vi "tm423_dualcamerasync.vi"() -> ()   [LabVIEW 2019]
panel:
  out "Camera Model":string
  out "Image":u16[][](graph)
  in  "capture":bool
  in  "Quit":bool
  out "Error Out":errorcluster {"code" format="%.0x"}
  # "This is an example of one way\nto synchronize two of the same\nmodel cameras."
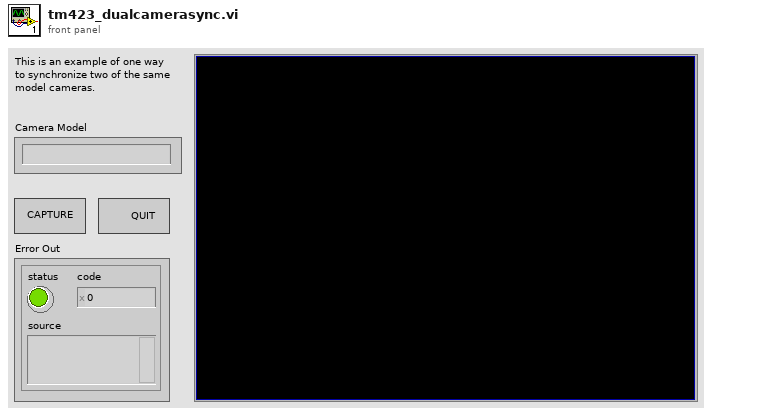
[diagram p1: front panel]
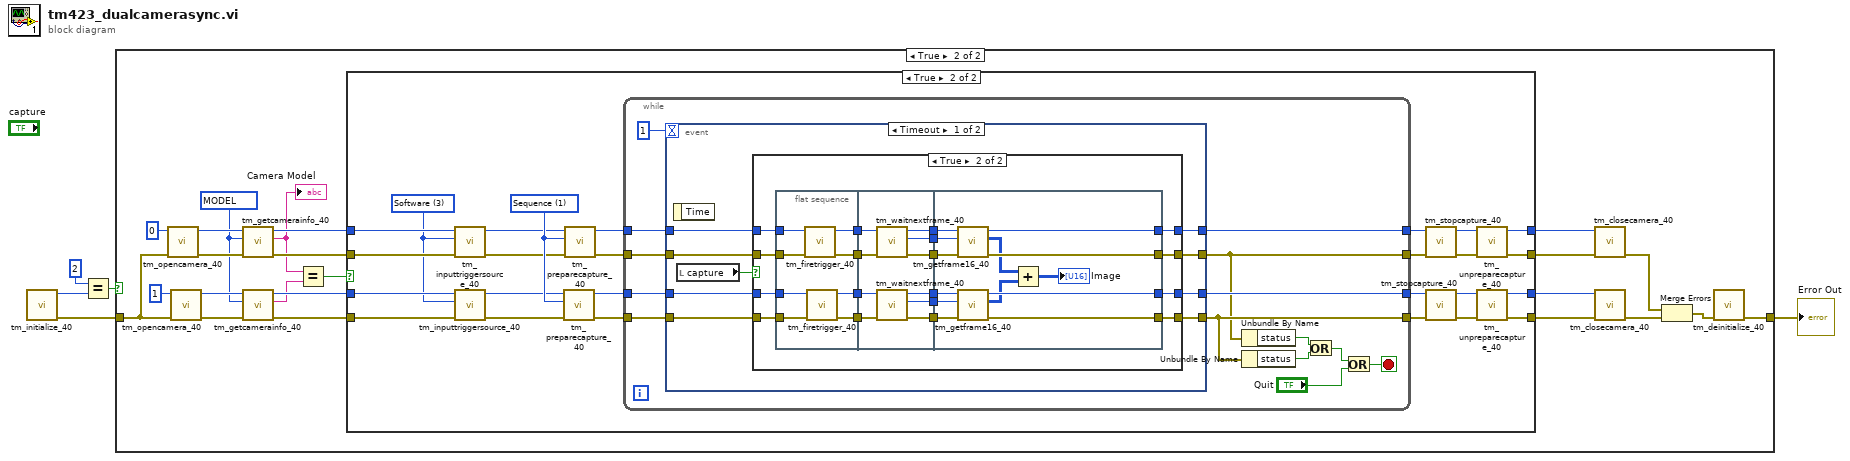
[diagram p0: block diagram]
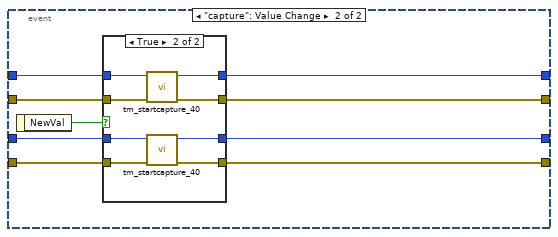
[diagram p5: hidden frame]
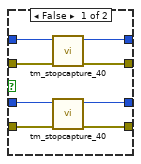
[diagram p6: hidden frame]
diagram:
  n1 = call <userlib>:"tm_initialize_40.vi"() -> ("error out"=w4:errorcluster, "Number Of Cameras"=w3:u32)  [unwired: 8 in, 2 out]
  n2 = Equal?(x=u32 2, y=w3) -> (x = y?=w1:bool)
  n3 = case shown="True" w1 {
    tunnel: w4 -> [w6 w26]
    tunnel: [w6 w28] -> w5
    frame False {
    }
    frame True {
      w18 = u32 67109124 items=["BUS"=67109121, "CAMERA ID"=67109122, "VENDOR"=67109123, "MODEL"=67109124, "CAMERA VERSION"=67109125, "DRIVER VERSION"=67109126, "MODULE VERSIOIN"=67109127, "DCAMAPI VERSION"=67109128] ("Info ID")
      n4 = call <userlib>:"tm_opencamera_40.vi"("error in (no error)"=w26, "Camera Index"=u32 0) -> ("error out"=w21:errorcluster, "Handle out"=w22:u32)  [unwired: 7 in, 1 out]
      n5 = call <userlib>:"tm_opencamera_40.vi"("error in (no error)"=w26, "Camera Index"=u32 1) -> ("error out"=w19:errorcluster, "Handle out"=w20:u32)  [unwired: 7 in, 1 out]
      n6 = call <userlib>:"tm_getcamerainfo_40.vi"("error in (no error)"=w21, "Info ID"=w18, "Handle in"=w22) -> ("error out"=w15:errorcluster, "String"=w9:string, "Handle out"=w14:u32)  [unwired: 6 in]
      "Camera Model" <- w9
      n7 = call <userlib>:"tm_getcamerainfo_40.vi"("error in (no error)"=w19, "Info ID"=w18, "Handle in"=w20) -> ("error out"=w16:errorcluster, "String"=w8:string, "Handle out"=w17:u32)  [unwired: 6 in]
      n8 = Equal?(x=w9, y=w8) -> (x = y?=w7:bool)
      n9 = case shown="True" w7 {
        tunnel: w17 -> [w33 w38]
        tunnel: w16 -> [w32 w37]
        tunnel: w15 -> [w31 w42]
        tunnel: w14 -> [w30 w41]
        tunnel: [w33 w50] -> w13
        tunnel: [w32 w49] -> w12
        tunnel: [w31 w47] -> w11
        tunnel: [w30 w48] -> w10
        frame False {
        }
        frame True {
          w34 = 3 items=["Internal"=1, "External"=2, "Software"=3, "Master Pulse"=4] ("Source")
          w51 = 1 items=["Snap", "Sequence"] ("Capture mode")
          n10 = call <userlib>:"tm_inputtriggersource_40.vi"("error in (no error)"=w42, "Source"=w34, "Handle in"=w41) -> ("error out"=w39:errorcluster, "Handle out"=w40:u32)  [unwired: 7 in]
          n11 = call <userlib>:"tm_inputtriggersource_40.vi"("error in (no error)"=w37, "Source"=w34, "Handle in"=w38) -> ("error out"=w35:errorcluster, "Handle out"=w36:u32)  [unwired: 7 in]
          n12 = call <userlib>:"tm_preparecapture_40.vi"("error in (no error)"=w35, "Capture mode"=w51, "Handle in"=w36) -> ("error out"=w43:errorcluster, "Handle out"=w44:u32)  [unwired: 5 in, 2 out]
          n13 = call <userlib>:"tm_preparecapture_40.vi"("error in (no error)"=w39, "Capture mode"=w51, "Handle in"=w40) -> ("error out"=w46:errorcluster, "Handle out"=w45:u32)  [unwired: 5 in, 2 out]
          n14 = while {
            tunnel: [w71] -> w59
            tunnel: [w65] -> w58
            tunnel: w44 -> [w73]
            tunnel: w43 -> [w72]
            tunnel: w45 -> [w68]
            tunnel: w46 -> [w67]
            tunnel: [w64] -> w52
            tunnel: [w66] -> w53
            stop <- w62 stop-if-true
            n15 = event shown="[0] Timeout" {
              selector: _ -> [_ _]
              dyn-events: _ -> [_ _]
              timeout: 1 -> [_ _]
              tunnel: w73 -> [w79 w143]
              tunnel: w72 -> [w78 w142]
              tunnel: [w75 w141] -> w71
              tunnel: [w74 w140] -> w65
              tunnel: w68 -> [w81 w139]
              tunnel: w67 -> [w80 w138]
              tunnel: [w76 w136] -> w66
              tunnel: [w77 w137] -> w64
              event Timeout {
                n16 = event-data() -> ()  [unwired: 1 in, 1 out]
                n17 = local read "capture"() -> (w82:bool)
                n18 = case shown="True" w82 {
                  tunnel: w81 -> [w86 w96]
                  tunnel: w80 -> [w85 w95]
                  tunnel: w79 -> [w83 w94]
                  tunnel: w78 -> [w84 w93]
                  tunnel: [w85 w92] -> w77
                  tunnel: [w86 w91] -> w76
                  tunnel: [w83 w90] -> w75
                  tunnel: [w84 w89] -> w74
                  frame False {
                  }
                  frame True {
                    n19 = flat-sequence {
                      tunnel: w94 -> [w112]
                      tunnel: w93 -> [w111]
                      tunnel: [w110] -> w104
                      tunnel: [w109] -> w103
                      tunnel: w96 -> [w108]
                      tunnel: [w106] -> w102
                      tunnel: w95 -> [w107]
                      tunnel: [w105] -> w101
                      tunnel: w104 -> [w119]
                      tunnel: w103 -> [w120]
                      tunnel: w102 -> [w121]
                      tunnel: w101 -> [w122]
                      tunnel: [w118] -> w100
                      tunnel: [w117] -> w99
                      tunnel: [w116] -> w98
                      tunnel: [w115] -> w97
                      tunnel: [w113] -> w88
                      tunnel: [w114] -> w87
                      tunnel: w100 -> [w134]
                      tunnel: w99 -> [w135]
                      tunnel: [w133] -> w91
                      tunnel: [w132] -> w92
                      tunnel: w98 -> [w131]
                      tunnel: w97 -> [w130]
                      tunnel: [w129] -> w90
                      tunnel: [w128] -> w89
                      tunnel: w88 -> [w127]
                      tunnel: w87 -> [w126]
                      frame #0 {
                        n20 = call <userlib>:"tm_firetrigger_40.vi"("error in (no error)"=w107, "Handle in"=w108) -> ("error out"=w105:errorcluster, "Handle out"=w106:u32)  [unwired: 8 in]
                        n21 = call <userlib>:"tm_firetrigger_40.vi"("error in (no error)"=w111, "Handle in"=w112) -> ("error out"=w109:errorcluster, "Handle out"=w110:u32)  [unwired: 8 in]
                      }
                      frame #1 {
                        n22 = call <userlib>:"tm_waitnextframe_40.vi"("error in (no error)"=w122, "Handle in"=w121) -> ("error out"=w117:errorcluster, "Frame Index"=w113:i32, "Handle out"=w118:u32)  [unwired: 6 in, 1 out]
                        n23 = call <userlib>:"tm_waitnextframe_40.vi"("error in (no error)"=w120, "Handle in"=w119) -> ("error out"=w115:errorcluster, "Frame Index"=w114:i32, "Handle out"=w116:u32)  [unwired: 6 in, 1 out]
                      }
                      frame #2 {
                        n24 = call <userlib>:"tm_getframe16_40.vi"("error in (no error)"=w135, "Frame Index"=w127, "Handle in"=w134) -> ("error out"=w132:errorcluster, "Data"=w125:u16[][], "Handle out"=w133:u32)  [unwired: 5 in, 1 out]
                        n25 = call <userlib>:"tm_getframe16_40.vi"("error in (no error)"=w130, "Frame Index"=w126, "Handle in"=w131) -> ("error out"=w128:errorcluster, "Data"=w124:u16[][], "Handle out"=w129:u32)  [unwired: 5 in, 1 out]
                        n26 = Add(x=w125, y=w124) -> (x+y=→"Image":u16[][])
                      }
                    }
                  }
                }
              }
              event "capture": Value Change {
                n27 = event-data() -> ("NewVal"=w144:bool)  [unwired: 1 in]
                n28 = case shown="True" w144 {
                  tunnel: w143 -> [w152 w160]
                  tunnel: w142 -> [w151 w159]
                  tunnel: [w150 w158] -> w141
                  tunnel: [w149 w157] -> w140
                  tunnel: w139 -> [w147 w156]
                  tunnel: w138 -> [w148 w155]
                  tunnel: [w146 w154] -> w136
                  tunnel: [w145 w153] -> w137
                  frame False {
                    n29 = call <userlib>:"tm_stopcapture_40.vi"("error in (no error)"=w148, "Handle in"=w147) -> ("error out"=w145:errorcluster, "Handle out"=w146:u32)  [unwired: 8 in]
                    n30 = call <userlib>:"tm_stopcapture_40.vi"("error in (no error)"=w151, "Handle in"=w152) -> ("error out"=w149:errorcluster, "Handle out"=w150:u32)  [unwired: 8 in]
                  }
                  frame True {
                    n31 = call <userlib>:"tm_startcapture_40.vi"("error in (no error)"=w155, "Handle in"=w156) -> ("error out"=w153:errorcluster, "Handle out"=w154:u32)  [unwired: 8 in]
                    n32 = call <userlib>:"tm_startcapture_40.vi"("error in (no error)"=w159, "Handle in"=w160) -> ("error out"=w157:errorcluster, "Handle out"=w158:u32)  [unwired: 8 in]
                  }
                }
              }
            }
            n33 = Unbundle By Name(w64) -> ("status"=w70:bool)
            n34 = Unbundle By Name(w65) -> ("status"=w63:bool)
            n35 = Or(x=w70, y=w63) -> (x .or. y?=w61:bool)
            n36 = Or(x=w61, y="Quit") -> (x .or. y?=w62:bool)
          }
          n37 = call <userlib>:"tm_stopcapture_40.vi"("error in (no error)"=w52, "Handle in"=w53) -> ("error out"=w54:errorcluster, "Handle out"=w55:u32)  [unwired: 8 in]
          n38 = call <userlib>:"tm_stopcapture_40.vi"("error in (no error)"=w58, "Handle in"=w59) -> ("error out"=w56:errorcluster, "Handle out"=w57:u32)  [unwired: 8 in]
          n39 = call <userlib>:"tm_unpreparecapture_40.vi"("error in (no error)"=w54, "Handle in"=w55) -> ("error out"=w47:errorcluster, "Handle out"=w48:u32)  [unwired: 8 in]
          n40 = call <userlib>:"tm_unpreparecapture_40.vi"("error in (no error)"=w56, "Handle in"=w57) -> ("error out"=w49:errorcluster, "Handle out"=w50:u32)  [unwired: 8 in]
        }
      }
      n41 = call <userlib>:"tm_closecamera_40.vi"("error in (no error)"=w11, "Handle in"=w10) -> ("error out"=w25:errorcluster)  [unwired: 9 in]
      n42 = call <userlib>:"tm_closecamera_40.vi"("error in (no error)"=w12, "Handle in"=w13) -> ("error out"=w24:errorcluster)  [unwired: 9 in]
      n43 = Merge Errors(w25, w24) -> (w23:errorcluster)
      n44 = call <userlib>:"tm_deinitialize_40.vi"("error in (no error)"=w23) -> ("error out"=w28:errorcluster)  [unwired: 10 in]
    }
  }
  "Error Out" <- w5
